vi "GT_BufGear.vi"(6 "fifo":i16, 8 "pos":i32, 9 "gearAxis":i16, 10 "crd":i16, 11 "rtn_In":cluster{"rtn":i16, "Func":string}) -> (0 "pos out":i32, 1 "gearAxis out":i16, 2 "crd out":i16, 3 "rtn_Out":cluster{"rtn":i16, "Func":string}, 4 "fifo out":i16)   [LabVIEW 2014]
uses:
  VC6/gts.dll
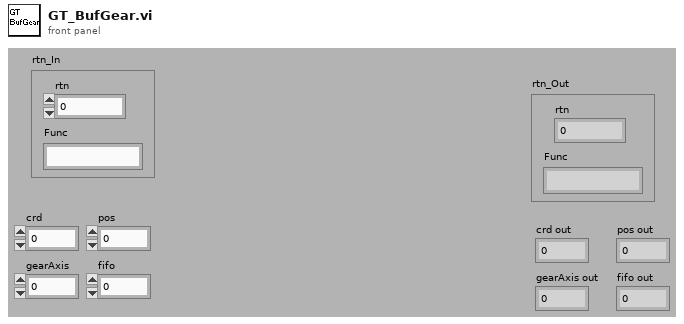
[diagram p1: front panel]
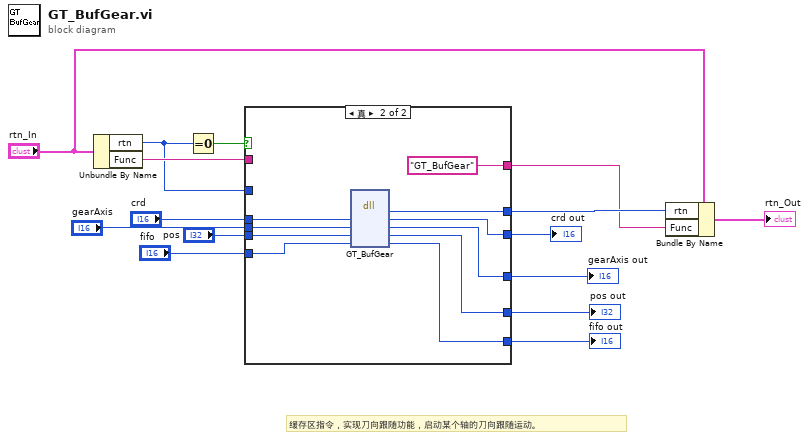
[diagram p0: block diagram]
diagram:
  # "缓存区指令，实现刀向跟随功能，启动某个轴的刀向跟随运动。"
  n1 = Unbundle By Name("rtn_In") -> ("rtn"=w1:i16, "Func"=w2:string)
  n2 = Equal To 0?(x=w1) -> (x = 0?=w15:bool)
  n3 = case shown="真" w15 {
    tunnel: [w20 w31] -> w12
    tunnel: [w21 "GT_BufGear" ("Func")] -> w11
    tunnel: "crd" -> [w19 w29]
    tunnel: "gearAxis" -> [w18 w28]
    tunnel: "pos" -> [w17 w27]
    tunnel: "fifo" -> [w16 w26]
    tunnel: [w19 w25] -> w6
    tunnel: [w18 w24] -> w5
    tunnel: [w17 w23] -> w4
    tunnel: [w16 w22] -> w3
    tunnel: w2 -> [w21 _]
    tunnel: w1 -> [w20 _]
    frame False {
    }
    frame True {
      n4 = dll-call lib="PTH2Fabs DNewGTS AC-800LWin7版源程序-20170926gts85VC6gts.dll" fn="GT_BufGear"("crd"=w29, "gearAxis"=w28, "pos"=w27, "fifo"=w26) -> ("rtn"=w31:i16, "crd"=w25:i16, "gearAxis"=w24:i16, "pos"=w23:i32, "fifo"=w22:i16)  [unwired: 3 in, 2 out]
    }
  }
  "crd out" <- w6
  "gearAxis out" <- w5
  "pos out" <- w4
  "fifo out" <- w3
  n5 = Bundle By Name(cluster="rtn_In", "rtn"=w12, "Func"=w11) -> (→"rtn_Out":cluster{"rtn":i16, "Func":string})
